vi "NMRvme1.vi"() -> ()   [LabVIEW 2013]
uses:
  <vilib>/Utility/file.llb/Read From Spreadsheet File (DBL).vi
  <vilib>/Analysis/NI_AALBase.lvlib
panel:
  in  "IF / LOG":bool
  in  "Q curve file":string="realback213.txt"
  out "File name 2":string="C:\\users\\plm\\Desktop\\rssmt\\realback213.txt"
  in  "AutoBaseline":bool=TRUE
  out "RF OK":bool=TRUE
  out "Peak area (V-MHz)":sgl=0.008127889 format="%.3f"
  in  "Gauss Fit":bool=TRUE
  out "NMR Graph + Fit":cluster{cluster{dbl, "Numeric":dbl}[]}[](graph)=[{[{224.37, "Numeric"=-0.04145357142857144}, {224.372, "Numeric"=-0.012618000000000315}, {224.374, "Numeric"=0.0017175714285717204}, {224.376, "Numeric"=0.013153142857142837}, {224.37800000000001, "Numeric"=0.014188714285713956}, {224.38, "Numeric"=0.00462428571428599}, {224.382, "Numeric"=0.010659857142857105}, {224.38400000000001, "Numeric"=0.013995428571428223}, {224.386, "Numeric"=0.009831000000000256}, {224.388, "Numeric"=0.0020665714285713747}, {224.39000000000001, "Numeric"=0.008202142857142491}, {224.392, "Numeric"=0.006637714285714524}, {224.394, "Numeric"=-0.003826714285714358}, {224.39600000000002, "Numeric"=0.0031088571428567586}, {224.398, "Numeric"=0.00814442857142879}, {224.4, "Numeric"=0.006579999999999907}, {224.40200000000002, "Numeric"=-0.0006844285714289766}, {224.404, "Numeric"=-0.0013488571428569435}, {224.406, "Numeric"=0.0024867142857141742}, {224.40800000000002, "Numeric"=-0.0009777142857147086}, {224.41, "Numeric"=-0.00034214285714267317}, {224.412, "Numeric"=0.003593428571428444}, {224.41400000000002, "Numeric"=-0.003471000000000441}, {224.416, "Numeric"=-0.011935428571428406}, {224.418, "Numeric"=-0.010899857142857293}, {224.42000000000002, "Numeric"=-0.0031642857142861734}, {224.422, "Numeric"=-0.00622871428571414}, {224.424, "Numeric"=-0.0077931428571430235}, {224.426, "Numeric"=-0.004857571428570988}, {224.428, "Numeric"=0.0015780000000001277}, {224.43, "Numeric"=-0.002886428571428756}, {224.432, "Numeric"=-0.0017508571428567236}, {224.434, "Numeric"=0.0026847142857143944}, {224.436, "Numeric"=0.007420285714285512}, {224.438, "Numeric"=0.0027558571428575466}, {224.44, "Numeric"=0.011991428571428661}, {224.442, "Numeric"=0.02662699999999978}, {224.444, "Numeric"=0.02006257142857181}, {224.446, "Numeric"=0.02129814285714293}, {224.448, "Numeric"=0.037033714285714045}, {224.45, "Numeric"=0.05596928571428608}, {224.452, "Numeric"=0.062004857142857195}, {224.454, "Numeric"=0.08174042857142831}, {224.456, "Numeric"=0.10687600000000036}, {224.458, "Numeric"=0.14241157142857147}, {224.46, "Numeric"=0.1791471428571426}, {224.462, "Numeric"=0.22848271428571462}, {224.464, "Numeric"=0.29191828571428574}, {224.466, "Numeric"=0.3412538571428569}, {224.468, "Numeric"=0.3747894285714289}, {224.47, "Numeric"=0.381525}, {224.472, "Numeric"=0.3590605714285711}, {224.474, "Numeric"=0.3070961428571431}, {224.476, "Numeric"=0.25393171428571426}, {224.478, "Numeric"=0.2103672857142854}, {224.48, "Numeric"=0.16230285714285742}, {224.482, "Numeric"=0.12513842857142854}, {224.484, "Numeric"=0.10307399999999965}, {224.486, "Numeric"=0.09000957142857167}, {224.488, "Numeric"=0.0641451428571428}, {224.49, "Numeric"=0.048880714285713917}, {224.492, "Numeric"=0.04641628571428595}, {224.494, "Numeric"=0.04145185714285707}, {224.496, "Numeric"=0.026187428571428188}, {224.498, "Numeric"=0.01932300000000022}, {224.5, "Numeric"=0.011758571428571335}, {224.502, "Numeric"=0.013594142857142454}, {224.504, "Numeric"=0.004529714285714487}, {224.506, "Numeric"=0.003165285714285603}, {224.508, "Numeric"=0.012300857142856721}, {224.51, "Numeric"=0.008136428571428754}, {224.512, "Numeric"=-0.0010280000000001293}, {224.514, "Numeric"=0.008307571428570987}, {224.516, "Numeric"=0.0028431428571430205}, {224.518, "Numeric"=-0.003921285714285863}, {224.51999999999998, "Numeric"=-0.00798571428571383}, {224.522, "Numeric"=0.0014498571428572884}, {224.524, "Numeric"=-0.010914571428571593}, {224.52599999999998, "Numeric"=-0.012578999999999561}, {224.528, "Numeric"=-0.005843428571428442}, {224.53, "Numeric"=-0.004707857142857326}, {224.53199999999998, "Numeric"=-0.005772285714285294}, {224.534, "Numeric"=-0.0037367142857141753}, {224.536, "Numeric"=-0.004801142857143059}, {224.53799999999998, "Numeric"=0.0018344285714289748}, {224.54, "Numeric"=-0.002029999999999909}, {224.542, "Numeric"=-0.0012944285714287934}, {224.54399999999998, "Numeric"=-0.0022588571428567585}, {224.546, "Numeric"=0.00047671428571435933}, {224.548, "Numeric"=-0.004687714285714524}, {224.54999999999998, "Numeric"=0.0016478571428575083}, {224.552, "Numeric"=0.012283428571428626}, {224.554, "Numeric"=0.001718999999999742}, {224.55599999999998, "Numeric"=-0.005245428571428226}, {224.558, "Numeric"=0.007790142857142893}, {224.56, "Numeric"=0.013025714285714009}, {224.56199999999998, "Numeric"=0.012961285714286041}, {224.564, "Numeric"=0.00679685714285716}, {224.566, "Numeric"=0.005632428571428276}, {224.56799999999998, "Numeric"=0.0020680000000003113}, {224.57, "Numeric"=-0.002996428571428572}]}, {[{224.37, "Numeric"=5.2932825772870536e-30}, {224.372, "Numeric"=7.430420643115727e-29}, {224.374, "Numeric"=9.886097445967585e-28}, {224.376, "Numeric"=1.2466930518175635e-26}, {224.37800000000001, "Numeric"=1.4901066627004084e-25}, {224.38, "Numeric"=1.688100659486582e-24}, {224.382, "Numeric"=1.8126021381496574e-23}, {224.38400000000001, "Numeric"=1.8447172199219203e-22}, {224.386, "Numeric"=1.7794274304456916e-21}, {224.388, "Numeric"=1.626874027313418e-20}, {224.39000000000001, "Numeric"=1.4097780225938308e-19}, {224.392, "Numeric"=1.157899087110963e-18}, {224.394, "Numeric"=9.013923180630229e-18}, {224.39600000000002, "Numeric"=6.65089603368413e-17}, {224.398, "Numeric"=4.651249441886708e-16}, {224.4, "Numeric"=3.0830620697993e-15}, {224.40200000000002, "Numeric"=1.9369484878289322e-14}, {224.404, "Numeric"=1.153392277361868e-13}, {224.406, "Numeric"=6.509672994691696e-13}, {224.40800000000002, "Numeric"=3.4822862816238414e-12}, {224.41, "Numeric"=1.765602505577922e-11}, {224.412, "Numeric"=8.484857764069426e-11}, {224.41400000000002, "Numeric"=3.8647318102636535e-10}, {224.416, "Numeric"=1.6684658524655477e-09}, {224.418, "Numeric"=6.827134342859112e-09}, {224.42000000000002, "Numeric"=2.647785140684226e-08}, {224.422, "Numeric"=9.733077863885966e-08}, {224.424, "Numeric"=3.3911017445667386e-07}, {224.426, "Numeric"=1.119836472870754e-06}, {224.428, "Numeric"=3.505028565234574e-06}, {224.43, "Numeric"=1.0398044712433144e-05}, {224.432, "Numeric"=2.923714522243014e-05}, {224.434, "Numeric"=7.791864914045631e-05}, {224.436, "Numeric"=0.00019682081682993705}, {224.438, "Numeric"=0.0004712201036484386}, {224.44, "Numeric"=0.0010693004670743202}, {224.442, "Numeric"=0.0022998465921726563}, {224.444, "Numeric"=0.004688362083048332}, {224.446, "Numeric"=0.009058714811436781}, {224.448, "Numeric"=0.016589572514090142}, {224.45, "Numeric"=0.028795655444229414}, {224.452, "Numeric"=0.047374201946661594}, {224.454, "Numeric"=0.07387202618318096}, {224.456, "Numeric"=0.10917954515304039}, {224.458, "Numeric"=0.15294163043161405}, {224.46, "Numeric"=0.20306417736124768}, {224.462, "Numeric"=0.2555430546998623}, {224.464, "Numeric"=0.30480214097820213}, {224.466, "Numeric"=0.34458400149733465}, {224.468, "Numeric"=0.36922863276623535}, {224.47, "Numeric"=0.37498923441221843}, {224.472, "Numeric"=0.3609652485192626}, {224.474, "Numeric"=0.32933292487381893}, {224.476, "Numeric"=0.28479218992475946}, {224.478, "Numeric"=0.23342327845566094}, {224.48, "Numeric"=0.1813357443171124}, {224.482, "Numeric"=0.13351985113898882}, {224.484, "Numeric"=0.09318187072642171}, {224.486, "Numeric"=0.06163681318055714}, {224.488, "Numeric"=0.03864311191710846}, {224.49, "Numeric"=0.02296292327375719}, {224.492, "Numeric"=0.01293318298129014}, {224.494, "Numeric"=0.006904096213229998}, {224.496, "Numeric"=0.0034932640397841662}, {224.498, "Numeric"=0.0016752481881938989}, {224.5, "Numeric"=0.0007614652101309337}, {224.502, "Numeric"=0.0003280530958967599}, {224.504, "Numeric"=0.00013395575628472308}, {224.506, "Numeric"=5.184439204744168e-05}, {224.508, "Numeric"=1.9018022504732002e-05}, {224.51, "Numeric"=6.612293057573541e-06}, {224.512, "Numeric"=2.1790239068025996e-06}, {224.514, "Numeric"=6.806048855678024e-07}, {224.516, "Numeric"=2.014889784011004e-07}, {224.518, "Numeric"=5.653673091391554e-08}, {224.51999999999998, "Numeric"=1.5036032524443308e-08}, {224.522, "Numeric"=3.790172580137738e-09}, {224.524, "Numeric"=9.055405021125294e-10}, {224.52599999999998, "Numeric"=2.0505952148424972e-10}, {224.528, "Numeric"=4.401241150373158e-11}, {224.53, "Numeric"=8.953514793612363e-12}, {224.53199999999998, "Numeric"=1.7263748941498657e-12}, {224.534, "Numeric"=3.1550034116253347e-13}, {224.536, "Numeric"=5.4649692193127713e-14}, {224.53799999999998, "Numeric"=8.972196420052746e-15}, {224.54, "Numeric"=1.3961529248709158e-15}, {224.542, "Numeric"=2.0591613298849692e-16}, {224.54399999999998, "Numeric"=2.878531077082073e-17}, {224.546, "Numeric"=3.813946851246364e-18}, {224.548, "Numeric"=4.78962504753706e-19}, {224.54999999999998, "Numeric"=5.701006830717959e-20}, {224.552, "Numeric"=6.431685084456173e-21}, {224.554, "Numeric"=6.877350330379831e-22}, {224.55599999999998, "Numeric"=6.970126965189061e-23}, {224.558, "Numeric"=6.695505881908243e-24}, {224.56, "Numeric"=6.09606049491365e-25}, {224.56199999999998, "Numeric"=5.260636643959879e-26}, {224.564, "Numeric"=4.302793549534568e-27}, {224.566, "Numeric"=3.335691493347872e-28}, {224.56799999999998, "Numeric"=2.4510062088406645e-29}, {224.57, "Numeric"=1.7069708739187154e-30}]}]
  in  "Amp of Q curve":dbl=1.7999999999999998 min=0.0 max=3.0 step=0.01 format="%_3f"
  in  "Subtract Q curve":bool
  in  "Adjust Tune":bool
  out "IF Offset":dbl(graph)=1.5808463999999993
  out "Pedestal Difference":dbl(graph)=0.00451
  out "# Good Spectra":i32=98
  in  "Quality cuts":bool=TRUE
  out "Pedestal OK":bool=TRUE
  out "Sweep #":i32=11
  out "1st Sweep":bool
  out "ADC volts OK":bool=TRUE
  out "Peak Height Distribution":cluster{"Y":dbl[], "Y":dbl[]}[](graph)=[{"Y"=[0.3573709171500425, 0.35765653573584955, 0.35794215432165655, 0.3582277729074636, 0.3585133914932706, 0.35879901007907766, 0.3590846286648847, 0.3593702472506917, 0.3596558658364988, 0.3599414844223058, 0.36022710300811284, 0.36051272159391984, 0.3607983401797269, 0.3610839587655339, 0.36136957735134095, 0.36165519593714796, 0.361940814522955, 0.362226433108762, 0.36251205169456907, 0.3627976702803761, 0.36308328886618313, 0.3633689074519902, 0.3636545260377972, 0.36394014462360424, 0.36422576320941125, 0.3645113817952183, 0.3647970003810253, 0.36508261896683236, 0.36536823755263936, 0.3656538561384464, 0.3659394747242534, 0.3662250933100605, 0.36651071189586754, 0.36679633048167454, 0.3670819490674816, 0.3673675676532886, 0.36765318623909565, 0.36793880482490265, 0.3682244234107097, 0.3685100419965167, 0.36879566058232377, 0.36908127916813077, 0.36936689775393783, 0.36965251633974483, 0.3699381349255519, 0.37022375351135894, 0.37050937209716595, 0.370794990682973, 0.37108060926878, 0.37136622785458706, 0.37165184644039406, 0.3719374650262011, 0.3722230836120081, 0.3725087021978152, 0.3727943207836222, 0.37307993936942924, 0.3733655579552363, 0.3736511765410433, 0.37393679512685035, 0.37422241371265735, 0.3745080322984644, 0.3747936508842714, 0.37507926947007847, 0.37536488805588547, 0.3756505066416925, 0.37593612522749953, 0.3762217438133066, 0.3765073623991136, 0.37679298098492064, 0.3770785995707277, 0.3773642181565347, 0.37764983674234176, 0.37793545532814876, 0.3782210739139558, 0.3785066924997628, 0.3787923110855699, 0.3790779296713769, 0.37936354825718394, 0.37964916684299094, 0.379934785428798, 0.380220404014605, 0.38050602260041205, 0.3807916411862191, 0.3810772597720261, 0.38136287835783317, 0.38164849694364017, 0.3819341155294472, 0.38221973411525423, 0.3825053527010613, 0.3827909712868683, 0.38307658987267534, 0.38336220845848235, 0.3836478270442894, 0.3839334456300964, 0.38421906421590346, 0.3845046828017105, 0.3847903013875175, 0.3850759199733246, 0.3853615385591316, 0.38564715714493863], "Y"=[1.0, 1.0, 0.0, 0.0, 0.0, 0.0, 0.0, 1.0, 0.0, 0.0, 0.0, 0.0, 0.0, 0.0, 1.0, 2.0, 0.0, 0.0, 0.0, 0.0, 0.0, 2.0, 1.0, 0.0, 0.0, 4.0, 3.0, 0.0, 1.0, 1.0, 2.0, 3.0, 1.0, 3.0, 4.0, 2.0, 1.0, 3.0, 1.0, 2.0, 0.0, 2.0, 4.0, 0.0, 3.0, 1.0, 2.0, 1.0, 1.0, 2.0, 2.0, 3.0, 3.0, 0.0, 1.0, 1.0, 2.0, 4.0, 4.0, 0.0, 2.0, 1.0, 2.0, 1.0, 0.0, 2.0, 1.0, 0.0, 1.0, 1.0, 2.0, 0.0, 0.0, 1.0, 2.0, 0.0, 1.0, 0.0, 0.0, 0.0, 1.0, 0.0, 0.0, 0.0, 1.0, 0.0, 1.0, 0.0, 0.0, 0.0, 0.0, 0.0, 0.0, 0.0, 0.0, 0.0, 0.0, 0.0, 0.0, 2.0]}]
  in  "# of Sweeps":i32=1000
  out "Std Dev (V)":dbl=0.0055525763936768 format="%_2g"
  out "Peak mean (V)":dbl=0.37047542021605057 format="%_4g"
  out "Peak Height":dbl(graph)=0.3754375514811412
  in  "Raw Data":bool=TRUE
  in  "Tank RF ON":bool=TRUE
  in  "IF Atten (dB)":i8 min=0 max=35 step=5
  in  "IFoffset (V)":dbl=1.5808463999999993 min=0.0 max=3000.0 step=0.001 format="%.4f"
  in  "Tune  (V)":dbl=1.057 min=0.0 max=5.0 step=0.001 format="%.4f"
  in  "Hi / Lo IF Gain":bool
  out "Voltage Array":sgl[](array[numeric])=[-0.0656, -0.0367, -0.0223, -0.0108, -0.0097, -0.0192, -0.0131, -0.0097, -0.0138, -0.0215, -0.0153, -0.0168, -0.0272, -0.0202, -0.0151, -0.0166, -0.0238, -0.0244, -0.0205, -0.0239, -0.0232, -0.0192, -0.0262, -0.0346, -0.0335, -0.0257, -0.0287, -0.0302, -0.0272, -0.0207, -0.0251, -0.0239, -0.0194, -0.0146, -0.0192, -0.0099, 0.0048, -0.0017, -0.0004, 0.0154, 0.0344, 0.0405, 0.0603, 0.0855, 0.1211, 0.1579, 0.2073, 0.2708, 0.3202, 0.3538, 0.3606, 0.3382, 0.2863, 0.2332, 0.1897, 0.1417, 0.1046, 0.0826, 0.0696, 0.0438, 0.0286, 0.0262, 0.0213, 0.0061, -0.0007, -0.0082, -0.0063, -0.0153, -0.0166, -0.0074, -0.0115, -0.0206, -0.0112, -0.0166, -0.0233, -0.0273, -0.0178, -0.0301, -0.0317, -0.0249, -0.0237, -0.0247, -0.0226, -0.0236, -0.0169, -0.0207, -0.0199, -0.0208, -0.018, -0.0231, -0.0167, -0.006, -0.0165, -0.0234, -0.0103, -0.005, -0.005, -0.0111, -0.0122, -0.0157, -0.0207] format="%.4f"
  in  "Invert Polarity":bool=TRUE
  out "Pedestal Diff (V)":sgl=0.00451 format="%.3f"
  out "Peak amp (V)":sgl=0.37543756 format="%.3f"
  in  "Save Data to File":bool=TRUE
  in  "RF Level (dBm)":dbl=-1.0 min=-10.0 max=1.0 step=0.1 format="%.2f"
  out "SMT error out":errorcluster
  out "Sample RMS (V)":dbl=0.009057425742574258 format="%.4f"
  in  "# Sample/step":i32=100 min=1 max=1000 step=100
  in  "ADC Rate (Hz)":i32=10000 min=1 max=20000 step=1000
  in  "ADC Range":i32(ring)=1 items=["+- 10 V"=1, "+- 2.5 V"=3]
  in  "Step Width (MHz)":dbl=0.002 min=0.0 max=1000.0 step=0.0005 format="%.4f"
  in  "Freq Span (MHz)":dbl=0.2 min=0.0 max=3000.0 step=0.1 format="%.3f"
  in  "Center Freq (MHz)":dbl=224.47 min=0.005 max=6000.0 step=0.1 format="%.3f"
  in  "Sweep Mode":u16(ring)=3 items=["Off", "Single", "Auto", "Step"]
  in  "GPIB Addr (28)":refnum<visa-resource-name>="GPIB0::28::INSTR"
  # "Settings"
  # "E1039 Prototype NMR Control Panel"
  # "D\nA\nC"
  # "R\nF\n\nG\ne\nn\ne\nr\na\nt\no\nr"
  # "A\nD\nC"
  # "D\na\nt\na"
  # "I\n/\nO"
  # "Results"
  # "A\nv\ne\nr\na\ng\ne"
  # "S\nw\ne\ne\np"
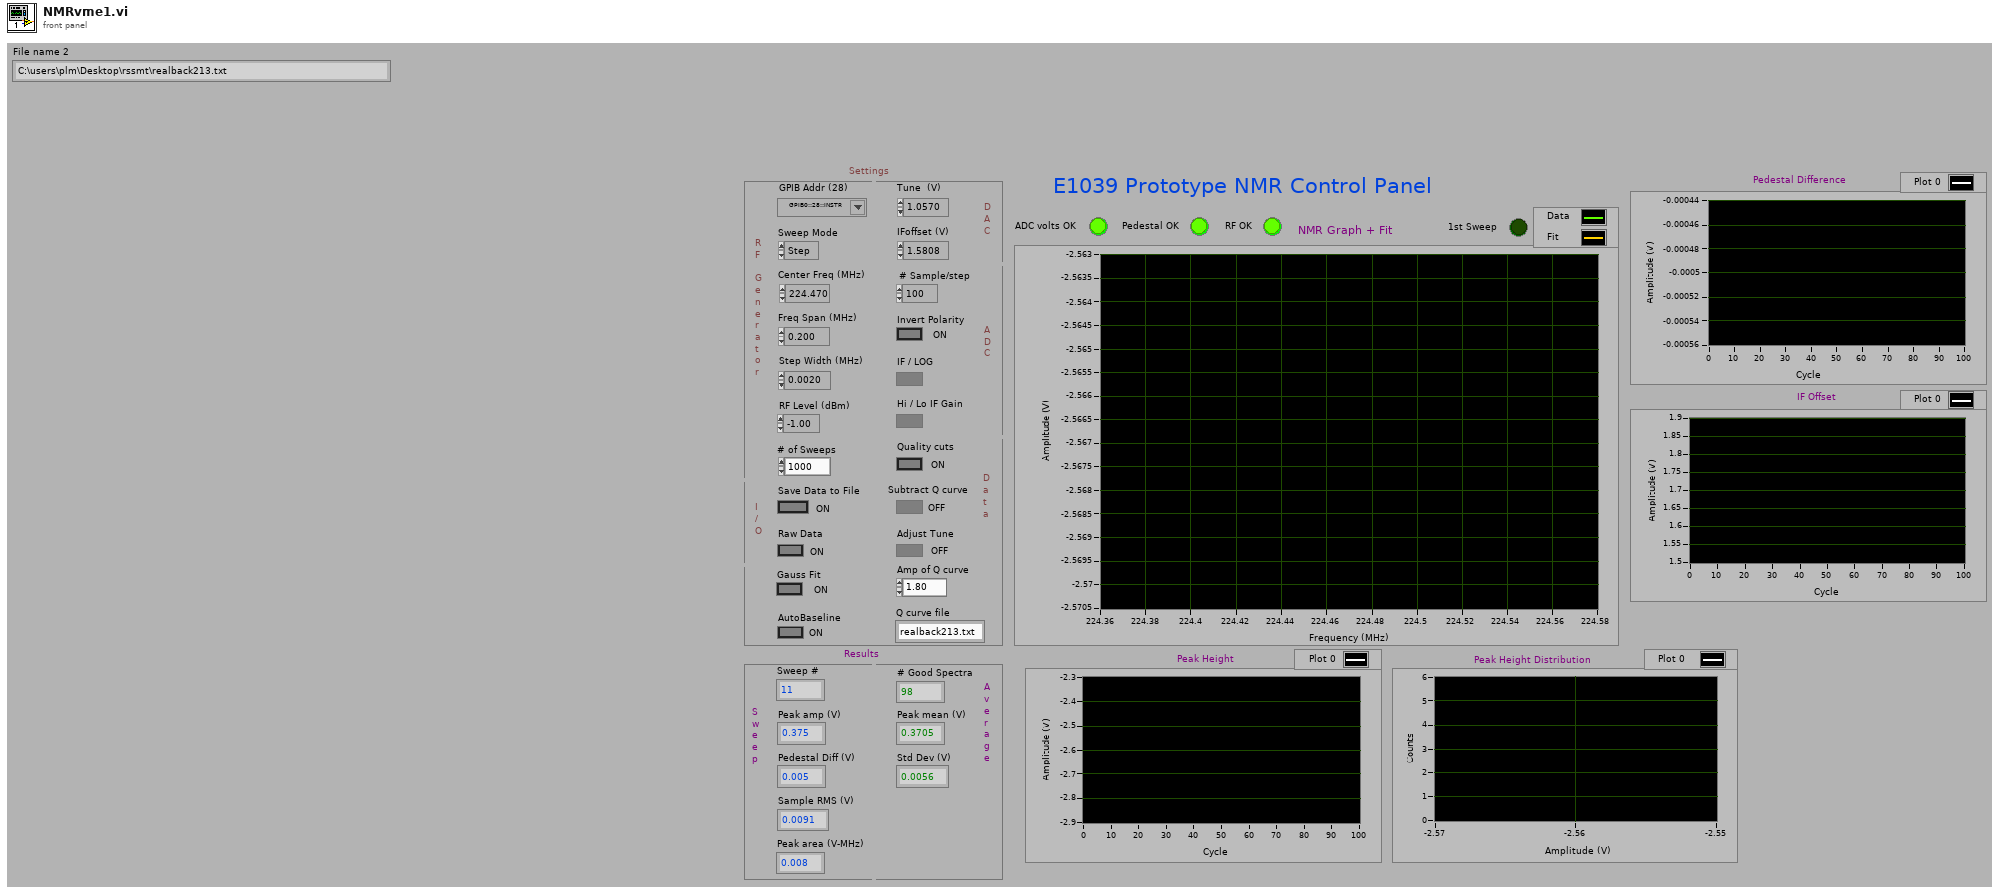
[diagram p1: front panel]
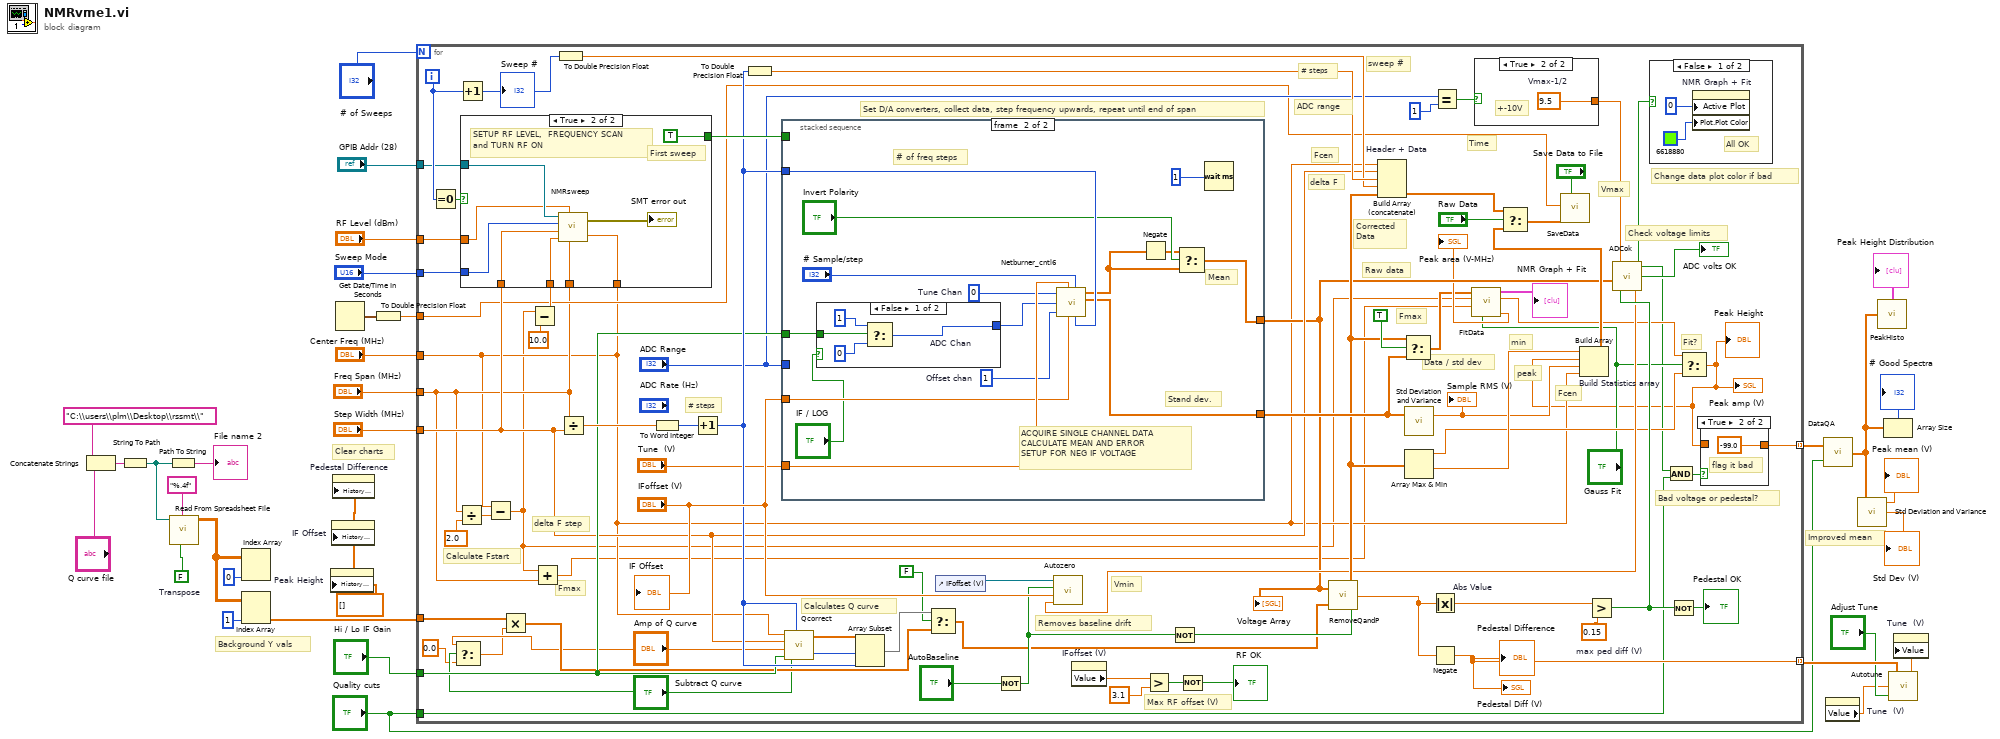
[diagram p0: block diagram]
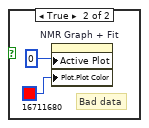
[diagram p2: hidden frame]
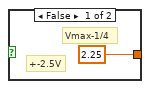
[diagram p3: hidden frame]
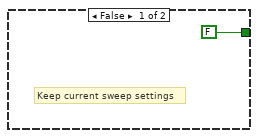
[diagram p5: hidden frame]
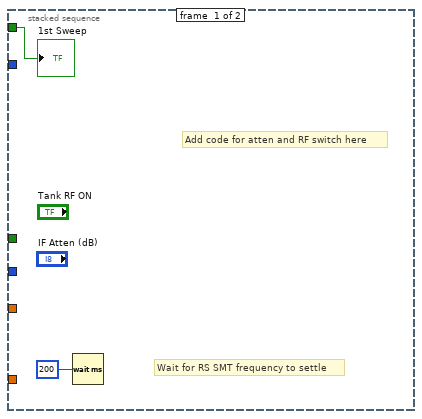
[diagram p6: hidden frame]
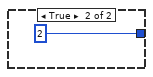
[diagram p7: hidden frame]
diagram:
  w8 = FALSE  # Transpose
  w17 = dbl[] []
  # "Background Y vals"
  # "Clear charts"
  # "Improved mean"
  n1 = Concatenate Strings "Concatenate Strings"("C:\\users\\plm\\Desktop\\rssmt\\", "Q curve file") -> (w11:string)
  n2 = String To Path(string=w11) -> (path=w7:path)
  n3 = Path To String(path=w7) -> (string=→"File name 2":string)
  n4 = call-poly <vilib>:"Read From Spreadsheet File.vi"("transpose (no:F)"=w8, "format (%.3f)"="%.4f", "file path (dialog if empty)"=w7) -> ("all rows"=w6:dbl[][])  [unwired: 4 in, 4 out]
  n5 = Index Array "Index Array"(array=w6, index (col)=0) -> ()  [unwired: 1 in, 1 out]
  n6 = Index Array(array=w6, index (col)=1) -> (element=w1:dbl[])  [unwired: 1 in]
  n7 = property on="Peak Height" class="WFChart (strict)"("History Data"=w17) -> ()  [unwired: 2 in, 2 out]
  n8 = property on="IF Offset" class="WFChart (strict)"("History Data"=w17) -> ()  [unwired: 2 in, 2 out]
  n9 = property on="Pedestal Difference" class="WFChart (strict)"("History Data"=w17) -> ()  [unwired: 2 in, 2 out]
  n10 = Get Date/Time In Seconds() -> (seconds since 1Jan1904=w13:timestamp)
  n11 = To Double Precision Float(number=w13) -> (double precision float=w12:dbl)
  n12 = for {
    N: "# of Sweeps" -> [_]
    tunnel: [w95] -> w29 mode=indexing
    tunnel: "Quality cuts" -> [w69]
    tunnel: [w78] -> w26 mode=indexing
    tunnel: "Center Freq (MHz)" -> [w56]
    tunnel: "Freq Span (MHz)" -> [w62]
    tunnel: "Step Width (MHz)" -> [w68]
    tunnel: "Sweep Mode" -> [w82]
    tunnel: "Hi / Lo IF Gain" -> [w81]
    tunnel: "GPIB Addr (28)" -> [w80]
    tunnel: "RF Level (dBm)" -> [w79]
    tunnel: w12 -> [w63]
    tunnel: w1 -> [w40]
    i -> [w93]
    w96 = 0.15  # max ped diff (V)
    # "Vmax"
    # "Change data plot color if bad"
    # "Max RF offset (V)"
    # "Fmax"
    # "Fit?"
    # "Fmax"
    # "Time"
    # "Vmin"
    # "min"
    # "peak"
    # "Raw data"
    # "Corrected\nData"
    # "Fcen"
    # "delta F"
    # "# steps"
    # "ADC range"
    # "sweep #"
    # "Fcen"
    # "Set D/A converters, collect data, step frequency upwards, repeat until end of span"
    # "Calculates Q curve"
    # "Removes baseline drift"
    # "Bad voltage or pedestal?"
    # "Check voltage limits"
    # "Data / std dev"
    # "# steps"
    # "Calculate Fstart"
    # "delta F step"
    n13 = Equal To 0?(x=w93) -> (x = 0?=w98:bool)
    n14 = Select(t="Amp of Q curve", s="Subtract Q curve", f=0.0) -> (s? t:f=w35:dbl)
    n15 = Divide(x=w62, y=sgl 2.0) -> (x/y=w109:dbl)
    n16 = Increment(x=w93) -> (x+1=w83:i32)
    "Sweep #" <- w83
    n17 = Subtract(x=w56, y=w109) -> (x-y=w51:dbl)
    n18 = Multiply(x=w40, y=w35) -> (x*y=w39:dbl[])
    n19 = Subtract(x=w51, y=10.0) -> (x-y=w107:dbl)
    n20 = case shown="True" w98 {
      tunnel: w107 -> [_ w129]
      tunnel: w68 -> [_ w127]
      tunnel: w56 -> [_ w126]
      tunnel: w62 -> [_ w128]
      tunnel: [FALSE TRUE] -> w97
      tunnel: w82 -> [_ w123]
      tunnel: w80 -> [_ w122]
      tunnel: w79 -> [_ w121]
      frame False {
        # "Keep current sweep settings"
      }
      frame True {
        # "First sweep"
        # "SETUP RF LEVEL,  FREQUENCY SCAN\nand TURN RF ON"
        n21 = call "NMRsweep.vi"("Center Freq (MHz)"=w126, "Freq Span (MHz)"=w128, "RF Level (dBm)"=w121, "Foffset (MHz)"=w129, "Step Width (MHz)"=w127, "Sweep Mode"=w123, "GPIB Addr (28)"=w122) -> ("error out"=→"SMT error out":errorcluster)
      }
    }
    n22 = Add(x=w51, y=w62) -> (x+y=w50:dbl)
    n23 = To Double Precision Float(number=w83) -> (double precision float=w84:dbl)
    n24 = Divide(x=w62, y=w68) -> (x/y=w111:dbl)
    n25 = To Word Integer(number=w111) -> (16bit integer=w108:i16)
    n26 = Increment(x=w108) -> (x+1=w87:i16)
    n27 = To Double Precision Float(number=w87) -> (double precision float=w86:dbl)
    n28 = stacked-sequence {
      tunnel: [_ w139] -> w101
      tunnel: [_ w137] -> w66
      tunnel: w87 -> [_ w142]
      tunnel: "IFoffset (V)" -> [_ w143]
      tunnel: w81 -> [_ w134]
      tunnel: w97 -> [w130 _]
      tunnel: "ADC Range" -> [_ _]
      tunnel: "Tune  (V)" -> [_ w144]
      frame #0 {
        # "Add code for atten and RF switch here"
        # "Wait for RS SMT frequency to settle"
        n29 = Wait (ms)(milliseconds to wait=200) -> ()  [unwired: 1 out]
        "1st Sweep" <- w130
      }
      frame #1 {
        w140 = 1  # Offset chan
        w141 = 0  # Tune Chan
        # "Stand dev."
        # "Mean"
        # "ACQUIRE SINGLE CHANNEL DATA\nCALCULATE MEAN AND ERROR\nSETUP FOR NEG IF VOLTAGE"
        # "# of freq steps"
        n30 = case shown="False" "IF / LOG" {
          tunnel: w134 -> [w150 _]
          tunnel: [w147 2] -> w133
          frame False {
            n31 = Select "ADC Chan"(t=1, s=w150, f=0) -> (s? t:f=w147:i32)
          }
          frame True {
          }
        }
        n32 = call "Netburner_cntl6.vi"("Tune DAC"=w141, "Tune Volt"=w144, "NMR ADC"=w133, "Offset DAC"=w140, "Offset Volt"=w143, "# Data"="# Sample/step", "# f steps"=w142) -> ("ADC value"=w136:dbl[], "ADC error"=w139:dbl[])  [unwired: 2 out]
        n33 = Negate(x=w136) -> (-x=w135:dbl[])
        n34 = Select(t=w135, s="Invert Polarity", f=w136) -> (s? t:f=w137:dbl[])
        n35 = Wait (ms)(milliseconds to wait=1) -> ()  [unwired: 1 out]
      }
    }
    "Voltage Array" <- w66
    n36 = call "Qcorrect.vi"("Subtract Q curve"="Subtract Q curve", "Nstep"=w87, "IF or Log"=w81, "Amp of Q curve"="Amp of Q curve", "Step Width (MHz)"=w68, "Center Freq (MHz)"=w56) -> ("Start"=w102:i32, "Array"=w103:dbl[])
    n37 = Array Subset "Array Subset"(array=w103, index=w102, length=w87) -> (w43:dbl[])
    n38 = Select(t=w43, s=FALSE, f=w39) -> (s? t:f=w42:dbl[])
    n39 = control-ref of="IFoffset (V)"() -> (w72:refnum<vi>)
    n40 = Not(x="AutoBaseline") -> (.not. x?=w45:bool)
    n41 = property on="IFoffset (V)" class="DigNum (strict)"() -> ("Value"=w60:dbl)  [unwired: 2 in, 2 out]
    n42 = Greater?(x=w60, y=3.1) -> (0:w58:bool)
    n43 = Not(x=w45) -> (.not. x?=w44:bool)
    n44 = Not(x=w58) -> (.not. x?=→"RF OK":bool)
    n45 = call "RemoveQandP.vi"("Raw data"=w66, "Qcurve"=w42, "Subtract Ped?"=w44) -> ("Corrected data"=w85:dbl[], "Ped L-R"=w89:dbl)
    n46 = Build Array (concatenate) "Header + Data"(w56, w68, w86, w84, w85) -> (w88:dbl[])
    n47 = Select(t=w85, s=TRUE, f=w101) -> (s? t:f=w52:dbl[])
    n48 = call <vilib>:"Std Deviation and Variance.vi"("X"=w101) -> ("mean"=w67:dbl)  [unwired: 1 in, 2 out]
    "Sample RMS (V)" <- w67
    n49 = Array Max & Min(array=w85) -> (max value=w61:dbl, min value=w100:dbl)  [unwired: 2 out]
    n50 = Absolute Value "Abs Value"(x=w89) -> (abs(x)=w91:dbl)
    n51 = Negate(x=w89) -> (-x=w78:dbl)
    "Pedestal Diff (V)" <- w78
    "Pedestal Difference" <- w78
    n52 = Equal?(x="ADC Range", y=1) -> (x = y?=w76:bool)
    n53 = call "FitData.vi"("Fit?"="Gauss Fit", "Fmax"=w50, "Fmin"=w51, "Yarray"=w52) -> ("Peak Area (V-MHz)"=→"Peak area (V-MHz)":dbl, "Amplitude (V)"=w54:dbl, "NMR Graph + Fit"=→"NMR Graph + Fit":cluster{cluster{dbl, "Numeric":dbl}[]}[])  [unwired: 2 out]
    n54 = case shown="True" w76 {
      tunnel: [2.25 w117] -> w73
      frame False {
        # "Vmax-1/4"
        # "+-2.5V"
      }
      frame True {
        w117 = 9.5  # Vmax-1/2
        # "+-10V"
      }
    }
    n55 = Greater?(x=w91, y=w96) -> (0:w77:bool)
    n56 = call "ADCok.vi"("PedOK"=w77, "Array"=w66, "Vmax-1/2"=w73) -> ("Vmin"=w71:dbl, "ADC voltages OK"=→"ADC volts OK":bool, "Allok"=w48:bool)
    n57 = call "Autozero.vi"("Vmin (V)"=w71, "IFoffset (V)"="IFoffset (V)", "IF or Log"=w45, "reference"=w72) -> ()
    n58 = case shown="False" w48 {
      frame False {
        # "All OK"
        n59 = property on="NMR Graph + Fit" class="XYGraph (strict)"("Active Plot"=0, "Plot.Plot Color"=u32 6618880) -> ()  [unwired: 2 in, 2 out]
      }
      frame True {
        # "Bad data"
        n60 = property on="NMR Graph + Fit" class="XYGraph (strict)"("Active Plot"=0, "Plot.Plot Color"=u32 16711680) -> ()  [unwired: 2 in, 2 out]
      }
    }
    n61 = And(x=w48, y=w69) -> (x .and. y?=w92:bool)
    n62 = Not(x=w77) -> (.not. x?=→"Pedestal OK":bool)
    n63 = Select(t=w54, s="Gauss Fit", f=w61) -> (s? t:f=w47:dbl)
    "Peak amp (V)" <- w47
    "Peak Height" <- w47
    n64 = Build Array "Build Statistics array"(w100, w47, w67, w56) -> (w106:dbl[])
    n65 = Select(t=w88, s="Raw Data", f=w106) -> (s? t:f=w64:dbl[])
    n66 = call "SaveData.vi"("Array"=w64, "Save Data to File"="Save Data to File", "Ext time (sec)"=w63) -> ()  [unwired: 1 out]
    n67 = case shown="True" w92 {
      tunnel: [w118 -99.0] -> w95
      tunnel: w47 -> [w118 _]
      frame False {
        # "Data OK"
      }
      frame True {
        # "flag it bad"
      }
    }
    "IF Offset" <- "IFoffset (V)"
  }
  n68 = call "DataQA.vi"("Quality cuts"="Quality cuts", "Data In"=w29) -> ("Data Out"=w28:dbl[])
  n69 = property on="Tune  (V)" class="DigNum (strict)"() -> ("Value"=w16:dbl)  [unwired: 2 in, 2 out]
  n70 = call <vilib>:"Std Deviation and Variance.vi"("X"=w28) -> ("mean"=→"Peak mean (V)":dbl, "standard deviation"=→"Std Dev (V)":dbl)  [unwired: 1 in, 1 out]
  n71 = call "PeakHisto.vi"("Data Out"=w28) -> ("XY Graph"=→"Peak Height Distribution":cluster{"Y":dbl[], "Y":dbl[]}[])
  n72 = Array Size(array=w28) -> (size(s)=→"# Good Spectra":i32)
  n73 = call "Autotune.vi"("Adjust Tune"="Adjust Tune", "Tune Vin"=w16, "Pedestal Diff"=w26) -> ("Tune Vout"=w15:dbl)
  n74 = property on="Tune  (V)" class="DigNum (strict)"("Value"=w15) -> ()  [unwired: 2 in, 2 out]
